vi "Client Info Loop.vi"(8 "error in (no error)":errorcluster, 11 "TCPMessaging in":refnum<class "TCPMessaging.lvclass">) -> (0 "error out":errorcluster)   [LabVIEW 2020, in "Vecto.lvlib" / "TCPMessaging.lvclass"]
doc: "Maintains the list of currently connected clients."
uses:
  TCPMessaging.lvclass
  Client Info Loop Data.ctl
  Connected Client.ctl
  Client Info.ctl
  TCPMessaging.lvclass/TCPMessaging.ctl
  <vilib>/Utility/miscctls.llb/LVMapReplaceAction.ctl
  VectoConfig/VectoConfig.lvlib
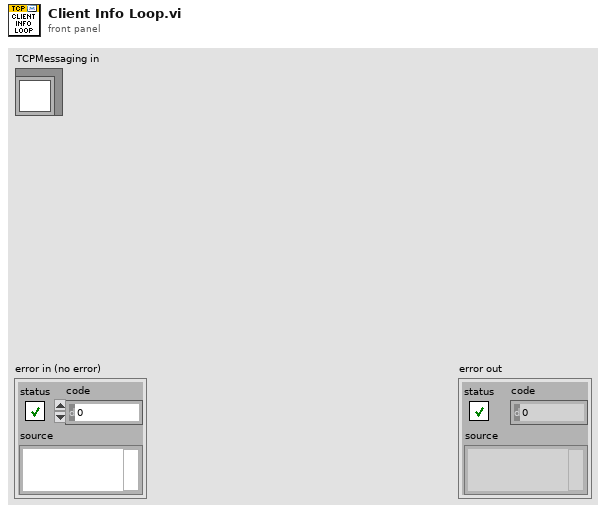
[diagram p1: front panel]
types:
  T1 = typedef "Vecto.lvlib/TCPMessaging.lvclass/Client Info Loop Data.ctl" = cluster{"Endpoint Map":map{string, T2}, "Node Map":map{u32, refnum<queue>[]}}
  T2 = typedef "Vecto.lvlib/TCPMessaging.lvclass/Connected Client.ctl" = cluster{"TCP":refnum<k5>, "Client Info":T3, "TX Q":refnum<queue>}
  T3 = typedef "VectoConfig.lvlib/Client Info.ctl" = cluster{"TcpClientHello":cluster{"node_id":u32, "system":string, "cluster":string, "node_name":string, "app_version":string, "config_version":string, "config_hash":string, "node_alias":string}, "Remote Address":string, "Remote Port":u16}
  T4 = typedef "LVMapReplaceAction.ctl" = enum32{"Modify Entry only if found", "Add or Modify Entry", "Delete Entry"}
  T5 = typedef "Vecto.lvlib/TCPMessaging.lvclass/Client Action Data.ctl" = cluster{"Client Action":T6, "Client Info":T3, "TCP":refnum<k5>, "TX Q":refnum<queue>}
  T6 = typedef "Vecto.lvlib/TCPMessaging.lvclass/Client Action.ctl" = enum16{"Connect", "Ready", "Disconnect"}
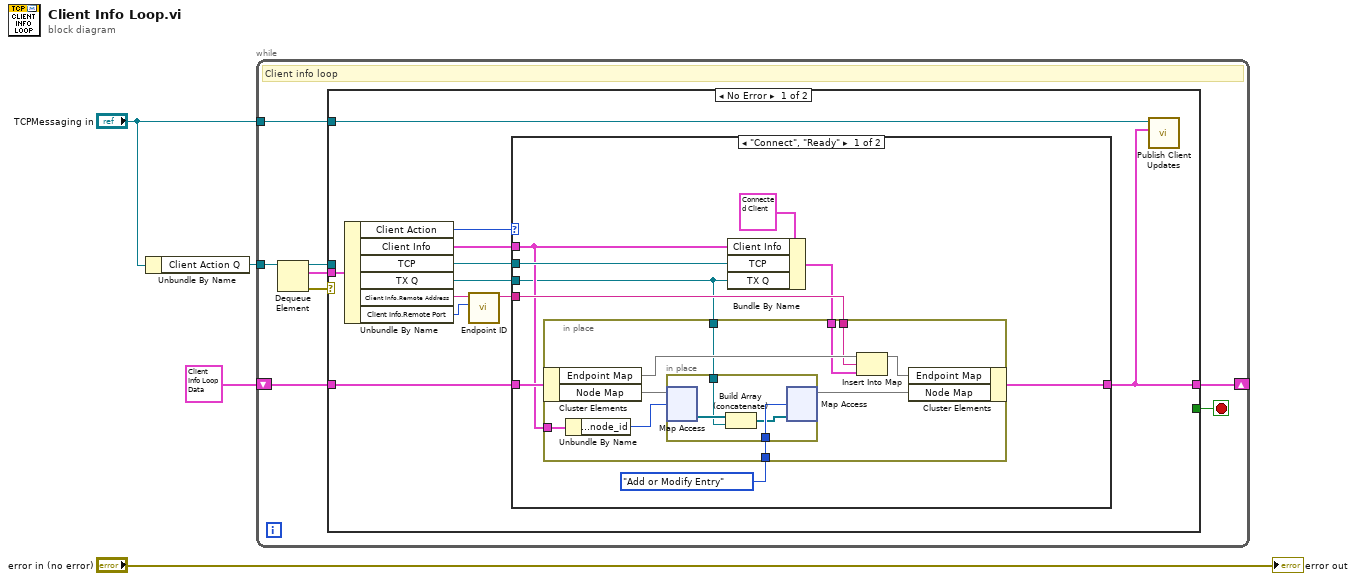
[diagram p0: block diagram]
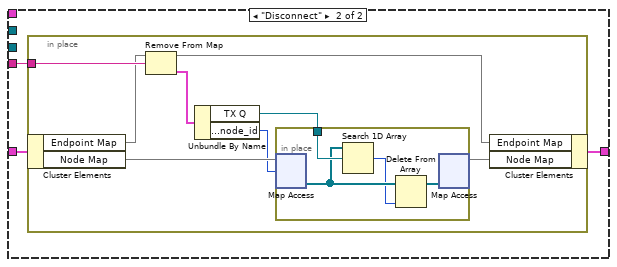
[diagram p2: hidden frame]
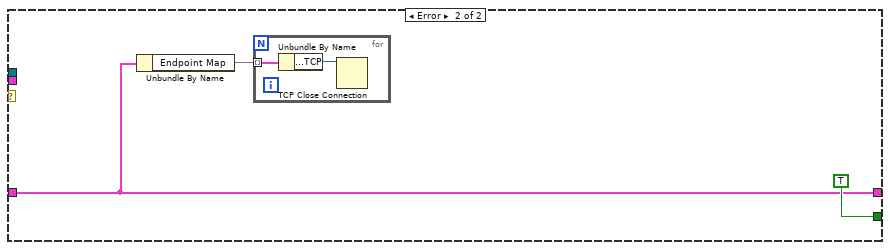
[diagram p3: hidden frame]
diagram:
  n1 = Unbundle By Name("TCPMessaging in") -> ("Client Action Q"=w2:refnum<queue>)
  n2 = while {
    tunnel: w2 -> [w12]
    shift-right: [w8] -> _
    shift-left: T1 {"Endpoint Map"={}, "Node Map"={}} ("Client Info Loop Data") -> [w9]
    tunnel: "TCPMessaging in" -> [w5]
    stop <- w7 stop-if-true
    # "Client info loop"
    n3 = Dequeue Element(queue=w12) -> (queue out=w6:refnum<queue>, element=w10:T5, error out=w11:errorcluster)  [unwired: 2 in, 1 out]
    n4 = case shown="No Error" w11 {
      tunnel: w10 -> [w23 _]
      tunnel: w9 -> [w18 w63]
      tunnel: [w14 w63] -> w8
      tunnel: [_ TRUE] -> w7
      tunnel: w6 -> [_ _]
      tunnel: w5 -> [w13 _]
      frame No Error {
        n5 = Unbundle By Name(w23) -> ("Client Action"=w20:T6, "Client Info"=w17:T3, "TCP"=w16:refnum<k5>, "TX Q"=w15:refnum<queue>, "Client Info.Remote Address"=w22:string, "Client Info.Remote Port"=w21:u16)
        n6 = call "Endpoint ID.vi"("Remote Port"=w21, "Remote Address"=w22) -> ("Endpoint ID"=w19:string)  [unwired: 9 in]
        n7 = case shown="\"Connect\", \"Ready\"" w20 {
          tunnel: w19 -> [w30 w47]
          tunnel: w18 -> [w32 w49]
          tunnel: [w31 w48] -> w14
          tunnel: w17 -> [w26 _]
          tunnel: w16 -> [w27 _]
          tunnel: w15 -> [w25 _]
          frame "Connect", "Ready" {
            n8 = Bundle By Name(cluster=T2 {"TCP"=refnum, "Client Info"={"TcpClientHello"={"node_id"=0, "system"="", "cluster"="", "node_name"="", "app_version"="", "config_version"="", "config_hash"="", "node_alias"=""}, "Remote Address"="", "Remote Port"=0}, "TX Q"=refnum} ("Connected Clients"), "Client Info"=w26, "TCP"=w27, "TX Q"=w25) -> (w28:T2)
            n9 = in-place {
              in-place-border: w30 -> [w41]
              in-place-border: w28 -> [w40]
              in-place-border: w26 -> [w37]
              in-place-border: w25 -> [w35]
              in-place-border: LVMapReplaceAction."Add or Modify Entry" ("action") -> [w33]
              n10 = in-place-cluster #1(w32) -> ("Endpoint Map"=w42:map{string, T2}, "Node Map"=w38:map{u32, refnum<queue>[]})
              n11 = Unbundle By Name(w37) -> ("TcpClientHello.node_id"=w36:u32)
              n12 = in-place {
                in-place-border: w35 -> [w45]
                in-place-border: w33 -> [w44]
                n13 = in-place-map #2(w38, w36) -> (w46:refnum<queue>[])  [unwired: 1 in, 1 out]
                n14 = Build Array (concatenate)(w46, w45) -> (w43:refnum<queue>[])
                n15 = in-place-map #2(w43, w44) -> (w34:map{u32, refnum<queue>[]})  [unwired: 2 out]
              }
              n16 = Insert Into Map(map in=w42, key=w41, value=w40) -> (map out=w39:map{string, T2})  [unwired: 2 out]
              n17 = in-place-cluster #1("Endpoint Map"=w39, "Node Map"=w34) -> (w31:T1)
            }
          }
          frame "Disconnect" {
            n18 = in-place {
              in-place-border: w47 -> [w57]
              n19 = in-place-cluster #3(w49) -> ("Endpoint Map"=w56:map{string, T2}, "Node Map"=w53:map{u32, refnum<queue>[]})
              n20 = Remove From Map(10:w57, 11:w56) -> (1:w54:T2, 3:w55:map{string, T2})  [unwired: 1 out]
              n21 = Unbundle By Name(w54) -> ("TX Q"=w50:refnum<queue>, "Client Info.TcpClientHello.node_id"=w52:u32)
              n22 = in-place {
                in-place-border: w50 -> [w61]
                n23 = in-place-map #4(w53, w52) -> (w60:refnum<queue>[])  [unwired: 1 in, 1 out]
                n24 = Search 1D Array(1D array=w60, element=w61) -> (index of element=w59:i32)  [unwired: 1 in]
                n25 = Delete From Array(array=w60, index=w59) -> (array with subset deleted=w58:refnum<queue>[])  [unwired: 1 in, 1 out]
                n26 = in-place-map #4(w58) -> (w51:map{u32, refnum<queue>[]})  [unwired: 1 in, 2 out]
              }
              n27 = in-place-cluster #3("Endpoint Map"=w55, "Node Map"=w51) -> (w48:T1)
            }
          }
        }
        n28 = call "Publish Client Updates.vi"("Client Info Loop Data"=w14, "TCPMessaging in"=w13) -> ()  [unwired: 8 in, 2 out]
      }
      frame Error {
        n29 = Unbundle By Name(w63) -> ("Endpoint Map"=w62:map{string, T2})
        n30 = for {
          tunnel: w62 -> [w66] mode=indexing
          n31 = Unbundle By Name(w66) -> ("Connected Client.TCP"=w65:refnum<k5>)
          n32 = TCP Close Connection(connection ID=w65) -> ()  [unwired: 2 in, 2 out]
        }
      }
    }
  }
  "error out" <- "error in (no error)"
